vi "TIO RPC Blocking_Ser.vi"(8 "error in (no error)":errorcluster, 9 "Payload":string, 10 "Named Method":string="mcu.desc", 11 "Nom de ressource VISA":refnum<visa-resource-name>) -> (0 "error out":errorcluster={"status"=TRUE, "code"=-1073807252, "source"="VISA Read in SLIP Decode Serial Read.vi->NN VISA Read.vi->NN RPC.vi"}, 1 "Response":bool, 2 "Respose":string, 3 "Nom de ressource VISA Out":refnum<visa-resource-name>)   [LabVIEW 2019]
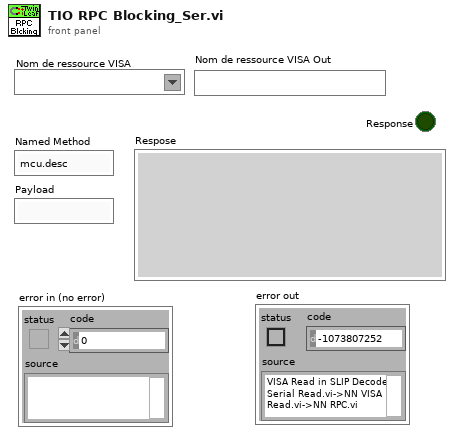
[diagram p1: front panel]
types:
  T1 = enum8{"Invalid", "Log", "RPC Request", "RPC Reply", "RPC Error", "Stream Description", "User"}
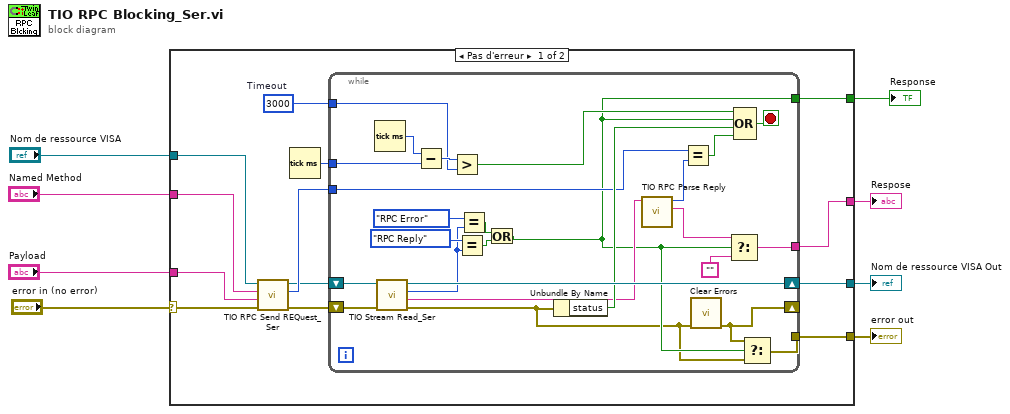
[diagram p0: block diagram]
diagram:
  n1 = case shown="Pas d'erreur" "error in (no error)" {
    selector: "error in (no error)" -> [w11 w48]
    tunnel: [w9 w48] -> w8
    tunnel: "Payload" -> [w20 _]
    tunnel: "Named Method" -> [w19 _]
    tunnel: [w17 _] -> w5
    tunnel: "Nom de ressource VISA" -> [w15 w49]
    tunnel: [w12 w49] -> w3
    tunnel: [w10 _] -> w1
    frame No Error {
      w13 = u32 3000  # Timeout
      n2 = call <userlib>:"TIO RPC Send REQuest_Ser.vi"("error in (no error)"=w11, "Payload"=w20, "Topic"=w19, "Nom de ressource VISA"=w15) -> ("error out"=w21:errorcluster, "Request ID"=w16:u16, "Nom de ressource VISA Out"=w14:refnum<visa-resource-name>)  [unwired: 5 in]
      n3 = Tick Count (ms)() -> (millisecond timer value=w18:u32)
      n4 = while {
        shift-right: [w23] -> _
        shift-left: w21 -> [w47]
        shift-right: [w46] -> w12
        shift-left: w14 -> [w26]
        tunnel: w18 -> [w44]
        tunnel: [w38] -> w17
        tunnel: w16 -> [w36]
        tunnel: w13 -> [w27]
        tunnel: [w24] -> w10
        tunnel: [w25] -> w9
        stop <- w40 stop-if-true
        n5 = Tick Count (ms)() -> (millisecond timer value=w45:u32)
        n6 = call <userlib>:"TIO Stream Read_Ser.vi"("error in (no error)"=w47, "VISA resource name"=w26) -> ("error out"=w22:errorcluster, "Payload"=w34:string, "Type"=w30:T1, "VISA resource name Out"=w46:refnum<visa-resource-name>)  [unwired: 5 in, 1 out]
        n7 = Subtract(x=w45, y=w44) -> (x-y=w43:u32)
        n8 = Greater?(x=w43, y=w27) -> (0:w42:bool)
        n9 = Equal?(x=T1."RPC Reply" ("Type"), y=w30) -> (x = y?=w28:bool)
        n10 = Equal?(x=T1."RPC Error" ("Type"), y=w30) -> (x = y?=w29:bool)
        n11 = Or(x=w29, y=w28) -> (x .or. y?=w24:bool)
        n12 = Unbundle By Name(w22) -> ("status"=w41:bool)
        n13 = call <userlib>:"TIO RPC Parse Reply.vi"("Payload"=w34) -> ("Payload"=w32:string, "Request ID"=w33:u16)  [unwired: 9 in]
        n14 = Equal?(x=w36, y=w33) -> (x = y?=w35:bool)
        n15 = call <vilib>:"Clear Errors.vi"("error in (no error)"=w22) -> ("error out"=w23:errorcluster)  [unwired: 5 in, 1 out]
        n16 = Select(t=w32, s=w24, f="") -> (s? t:f=w38:string)
        n17 = Compound Arithmetic op=OR(w42, w24, w41, w35) -> (w40:bool)
        n18 = Select(t=w23, s=w24, f=w22) -> (s? t:f=w25:errorcluster)
      }
    }
    frame Error {
    }
  }
  "error out" <- w8
  "Respose" <- w5
  "Nom de ressource VISA Out" <- w3
  "Response" <- w1
